vi "Load.vi"(8 "error in":errorcluster, 11 "Gantry in":refnum<class "Gantry Class.lvclass">) -> (0 "error out":errorcluster, 3 "PickerTool out":refnum<class "PickerTool Class.lvclass">)   [LabVIEW 2017, in "PickerTool Class.lvclass"]
uses:
  PickerTool Class.lvclass
  C:/Users/cfang/Desktop/pixel-gantry-control/Gantry/Shared Components/Gantry Class/Gantry Class.lvclass
  Gantry Class/Gantry Class.lvclass
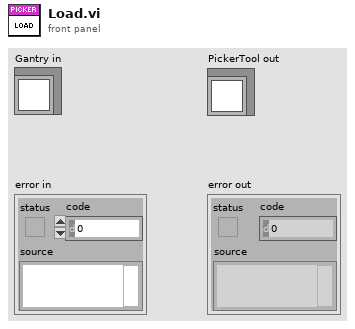
[diagram p1: front panel]
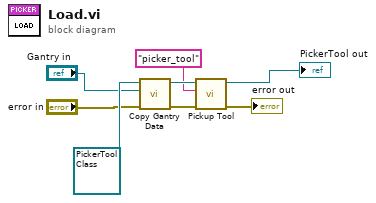
[diagram p0: block diagram]
diagram:
  n1 = call "Copy Gantry Data.vi"("error in"="error in", "Gantry Source"="Gantry in", "Gantry Dest"=refnum<class "PickerTool Class.lvclass"> refnum ("PickupTool Class in")) -> ("error out"=w7:errorcluster, "Gantry Result"=w8:refnum<class "PickerTool Class.lvclass">)  [unwired: 7 in]
  n2 = call-dynamic "Pickup Tool.vi"("error in"=w7, "Tool"="picker_tool", "Gantry in"=w8) -> ("error out"=→"error out":errorcluster, "Gantry out"=→"PickerTool out":refnum<class "PickerTool Class.lvclass">)  [unwired: 7 in]
